vi "remote path.vi"(9 "remote path":path, 10 "remote":bool, 11 "database":string="database1.mdb") -> (3 "appended path":path)   [LabVIEW 2016]
uses:
  <vilib>/Utility/sysdir.llb/System Directory Type.ctl
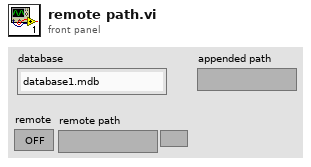
[diagram p1: front panel]
types:
  T1 = typedef "System Directory Type.ctl" = i32
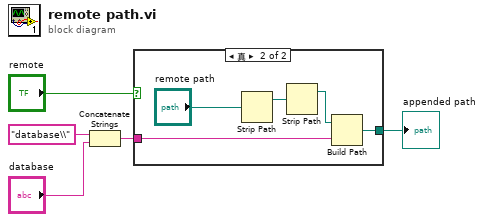
[diagram p0: block diagram]
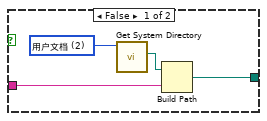
[diagram p2: hidden frame]
diagram:
  n1 = Concatenate Strings("database\\" ("名称或相对路径"), "database") -> (w4:string)
  n2 = case shown="真" "remote" {
    tunnel: w4 -> [w7 w13]
    tunnel: [w6 w11] -> w5
    frame False {
      w8 = T1 2 items=["用户目录"=0, "用户桌面"=1, "用户文档"=2, "用户应用程序数据"=3, "用户设置"=4, "用户临时目录"=5, "公共文档"=6, "公共应用程序数据"=7, "公共设置"=8, "公共缓存"=13, "系统核心库"=9, "系统安装库"=10, "应用程序文件"=11, "启动盘根目录"=12] ("system directory type")
      n3 = call <vilib>:"Get System Directory.vi"("system directory type"=w8) -> ("system directory"=w9:path)  [unwired: 10 in]
      n4 = Build Path(base path=w9, name or relative path=w7) -> (appended path=w6:path)
    }
    frame True {
      n5 = Strip Path(path="remote path") -> (stripped path=w14:path)  [unwired: 1 out]
      n6 = Strip Path(path=w14) -> (stripped path=w12:path)  [unwired: 1 out]
      n7 = Build Path(base path=w12, name or relative path=w13) -> (appended path=w11:path)
    }
  }
  "appended path" <- w5
